vi "RampKick.vi"(0 "Init (F)":bool, 4 "dt [s]":sgl, 5 "Output Max [unit]":sgl, 6 "Re-Kick Delay [s]":sgl, 7 "Output Min [unit]":sgl, 8 "Kick?":bool, 9 "Kick Magnitude [unit]":sgl, 10 "Offset [unit] (0)":sgl, 11 "Gain [unit/s]":sgl) -> (2 "Kicked":bool, 3 "Ramp/Kick Output":sgl)   [LabVIEW 2015, in "ECS-RT.lvlib"]
uses:
  ECS-RT.lvlib
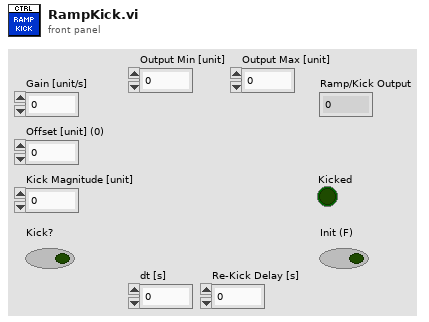
[diagram p1: front panel]
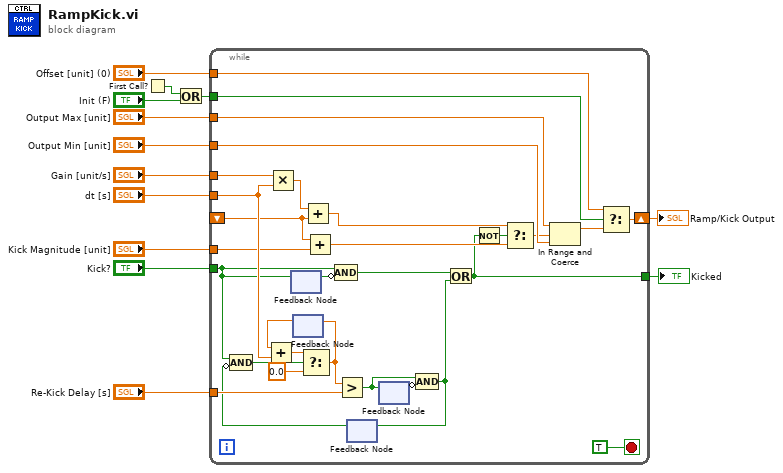
[diagram p0: block diagram]
diagram:
  n1 = First Call?() -> (First Call?: T/F=w2:bool)
  n2 = Or(x=w2, y="Init (F)") -> (x .or. y?=w4:bool)
  n3 = while {
    shift-right: [w21] -> w13
    shift-left: _ -> [w16]
    tunnel: "Output Max [unit]" -> [w43]
    tunnel: "Output Min [unit]" -> [w42]
    tunnel: "Gain [unit/s]" -> [w41]
    tunnel: "dt [s]" -> [w38]
    tunnel: "Kick?" -> [w26]
    tunnel: "Re-Kick Delay [s]" -> [w35]
    tunnel: "Kick Magnitude [unit]" -> [w33]
    tunnel: w4 -> [w20]
    tunnel: "Offset [unit] (0)" -> [w19]
    tunnel: [w14] -> w1
    stop <- TRUE stop-if-true
    n4 = Multiply(x=w41, y=w38) -> (x*y=w17:sgl)
    n5 = feedback #1() -> (w31:bool)  [unwired: 1 in]
    n6 = feedback-in #1(w26) -> ()
    n7 = feedback #2() -> (w39:sgl)  [unwired: 1 in]
    n8 = Add(x=w39, y=w38) -> (x+y=w40:sgl)
    n9 = Add(x=w17, y=w16) -> (x+y=w34:sgl)
    n10 = Add(x=w16, y=w33) -> (x+y=w32:sgl)
    n11 = Compound Arithmetic op=AND(w26, invert w31) -> (w30:bool)
    n12 = feedback #3() -> (w24:bool)  [unwired: 1 in]
    n13 = Compound Arithmetic op=AND(w26, invert w24) -> (w25:bool)
    n14 = Select(t=w40, s=w25, f=sgl 0.0) -> (s? t:f=w36:sgl)
    n15 = feedback-in #2(w36) -> ()
    n16 = Greater?(x=w36, y=w35) -> (0:w28:bool)
    n17 = feedback #4() -> (w29:bool)  [unwired: 1 in]
    n18 = feedback-in #4(w28) -> ()
    n19 = Compound Arithmetic op=AND(w28, invert w29) -> (w27:bool)
    n20 = feedback-in #3(w27) -> ()
    n21 = Or(x=w30, y=w27) -> (x .or. y?=w14:bool)
    n22 = Not(x=w14) -> (.not. x?=w15:bool)
    n23 = Select(t=w34, s=w15, f=w32) -> (s? t:f=w23:sgl)
    n24 = In Range and Coerce(upper limit=w43, x=w23, lower limit=w42) -> (coerced(x)=w22:sgl)  [unwired: 1 out]
    n25 = Select(t=w19, s=w20, f=w22) -> (s? t:f=w21:sgl)
  }
  "Ramp/Kick Output" <- w13
  "Kicked" <- w1
